vi "Get Command Bits.vi"(8 "error in (no error)":errorcluster, 11 "RFFE RegWriteExt Command in":refnum<class "RFFE RegWriteExt Command.lvclass">) -> (0 "error out":errorcluster, 2 "Command Bits":u8[](array[numeric]) format="%02x", 3 "RFFE RegWriteExt Command out":refnum<class "RFFE RegWriteExt Command.lvclass">)   [LabVIEW 2018, in "MIPI RFFE API.lvlib" / "RFFE RegWriteExt Command.lvclass"]
uses:
  RFFE RegWriteExt Command.lvclass
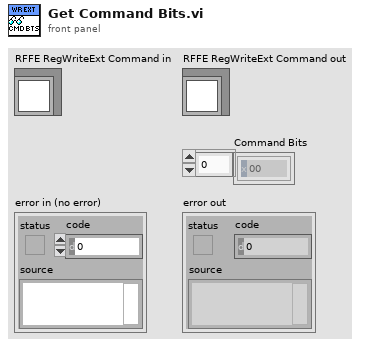
[diagram p1: front panel]
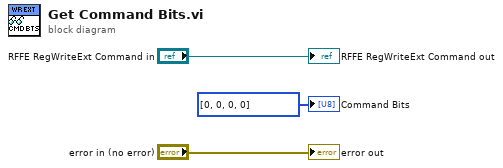
[diagram p0: block diagram]
diagram:
  "error out" <- "error in (no error)"
  "RFFE RegWriteExt Command out" <- "RFFE RegWriteExt Command in"
  "Command Bits" <- u8[] [0, 0, 0, 0] ("Command Bits")
